vi "rqp_Start Exiting.vi"(7 "Caller in":refnum<class "Worker.lvclass">, 8 "error in":errorcluster, 11 "UART Worker in":refnum<class "UART Worker.lvclass">) -> (0 "error out":errorcluster, 3 "dup UART Worker out":refnum<class "UART Worker.lvclass">, 5 "dup Caller out":refnum<class "Worker.lvclass">)   [LabVIEW 2020, in "UART Worker.lvclass"]
doc: "This VI will indirectly send a message to the <Start Exiting> MHL case of the Worker that own this VI.\n---\nThe shutdown sequence of the Worker that owns this VI will be initiated."
uses:
  UART Worker.lvclass
  <vilib>/addons/_Workers/Library/Classes/Worker/Worker.lvclass
  <vilib>/addons/_Workers/Library/Classes/Message Queue/Message Queue.lvclass
  UART Worker.lvclass/UART Worker.ctl
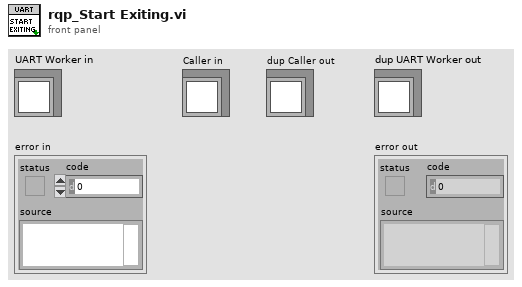
[diagram p1: front panel]
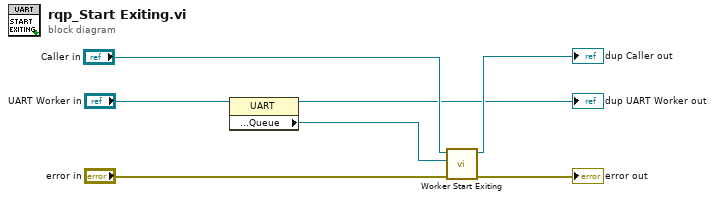
[diagram p0: block diagram]
diagram:
  n1 = property class="UART"(reference="UART Worker in") -> (reference out=→"dup UART Worker out":refnum<class "UART Worker.lvclass">, "Accessors:Read:Public API:Queue"=w1:refnum<class "Message Queue.lvclass">)  [unwired: 1 in, 1 out]
  n2 = call-dynamic "Worker Start Exiting.vi"("error_in"="error in", "Message Queue"=w1, "Worker"="Caller in") -> ("error out"=→"error out":errorcluster, "dup Worker out"=→"dup Caller out":refnum<class "Worker.lvclass">)  [unwired: 7 in]
